vi "SimpleReadWriteRead.vi"() -> ()   [LabVIEW 2017]
uses:
  <vilib>/express/express analysis/Spectral/Block/exnSpectralBlock spectral measurements RMS poly.vi
  <vilib>/express/express analysis/Spectral/Block/exnSpectralBlock spectral measurements RMS DDT.vi
  <vilib>/express/express analysis/Spectral/XNode/ExpressSpectralMeasurementsBlockNode.xnode
panel:
  in  "100 Hz high-pass":bool
  out "Waveform Graph 2":dynamicdata(graph)
  out "Waveform Graph":dynamicdata(graph)
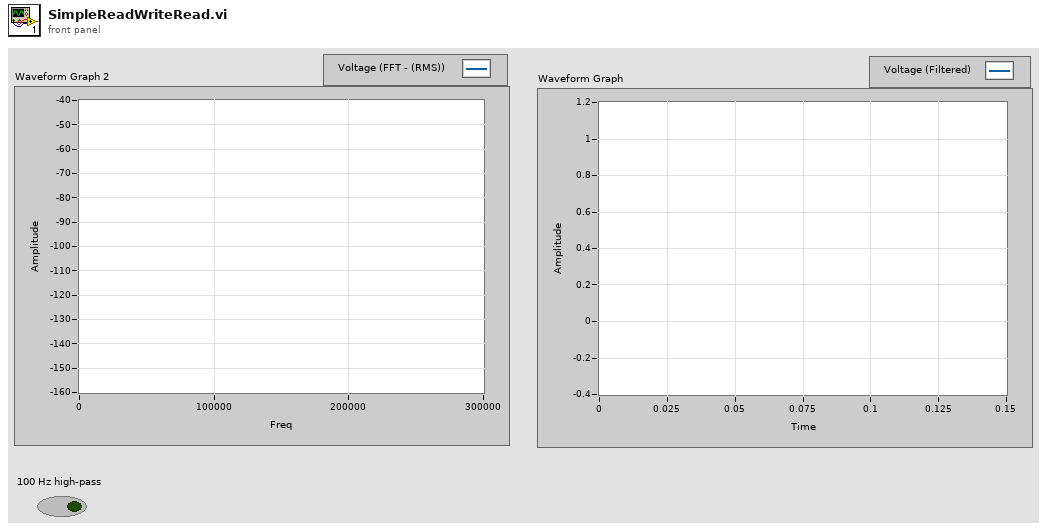
[diagram p1: front panel]
types:
  T1 = cluster{"averaging mode":u16, "weighting mode":u16, "number of averages":u32}
  T2 = cluster{"dB On (F)":bool, "unwrap phase (F)":bool, "convert to degree (F)":bool}
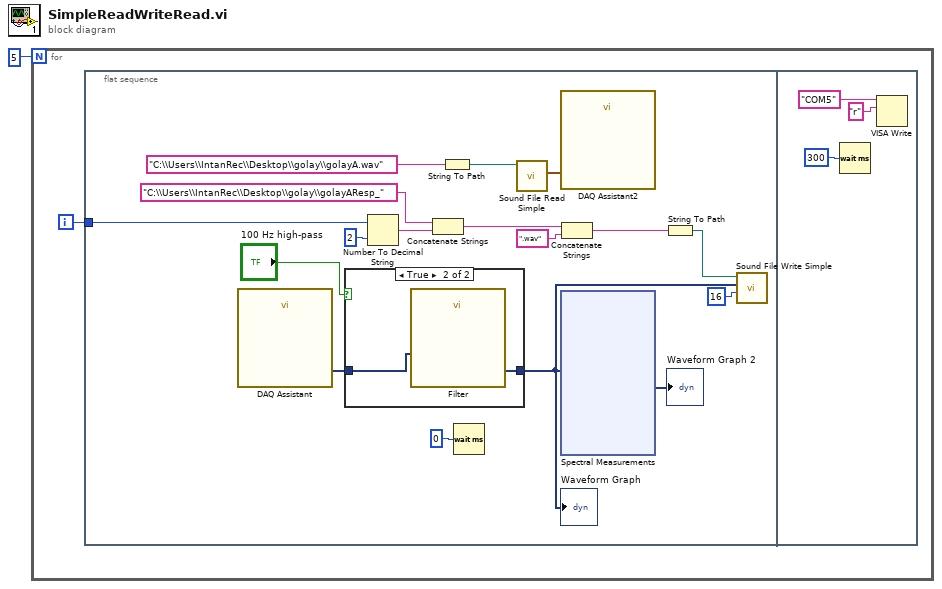
[diagram p0: block diagram]
diagram:
  n1 = for {
    N: 5 -> [_]
    i -> [w2]
    n2 = flat-sequence {
      tunnel: w2 -> [w14]
      frame #0 {
        n3 = call "DAQ Assistant"() -> ("data"=w8:dynamicdata)  [unwired: 17 in, 2 out]
        n4 = case shown="True" "100 Hz high-pass" {
          tunnel: w8 -> [w20 w22]
          tunnel: [w20 w21] -> w7
          frame False {
          }
          frame True {
            n5 = call "Filter"("Signal"=w22) -> ("Filtered Signal"=w21:dynamicdata)  [unwired: 9 in, 1 out]
          }
        }
        "Waveform Graph" <- w7
        n6 = Number To Decimal String(number=w14, width (-)=2) -> (decimal integer string=w12:string)
        n7 = Concatenate Strings("C:\\Users\\IntanRec\\Desktop\\golay\\golayAResp_", w12) -> (w11:string)
        n8 = String To Path(string="C:\\Users\\IntanRec\\Desktop\\golay\\golayA.wav") -> (path=w5:path)
        n9 = Wait (ms)(milliseconds to wait=0) -> ()  [unwired: 1 out]
        n10 = call <vilib>:"Sound File Read Simple.vi"("path"=w5) -> ("data"=w18:waveform(dbl)[])  [unwired: 7 in, 3 out]
        n11 = call "DAQ Assistant2"("data"=w18) -> ()  [unwired: 17 in, 2 out]
        n12 = xnode "Spectral Measurements"("Signals"=w7) -> ("FFT - (RMS)"=→"Waveform Graph 2":dynamicdata)  [unwired: 1 in, 2 out]
        n13 = Concatenate Strings(w11, ".wav") -> (w9:string)
        n14 = String To Path(string=w9) -> (path=w16:path)
        n15 = call <vilib>:"Sound File Write Simple.vi"("bits per sample"=16, "data"=w7, "path"=w16) -> ()  [unwired: 7 in, 2 out]
      }
      frame #1 {
        n16 = Wait (ms)(milliseconds to wait=300) -> ()  [unwired: 1 out]
        n17 = VISA Write(VISA resource name="COM5", write buffer="r") -> ()  [unwired: 1 in, 3 out]
      }
    }
  }
